vi "RT - Volume Track Math.vi"(10 "input cluster":T1={"Mute"=FALSE, "Solo"=FALSE, "Record"=FALSE, "Pan"=0.49531942166472487, "Volume"=0.0} {"Volume" scale=1.0..10.0; "Pan" scale=0.0..1.0}) -> (2 "Numeric":u16, 3 "Numeric 2":u16)   [LabVIEW 2014]
uses:
  Controls/Track Volume Settings.ctl
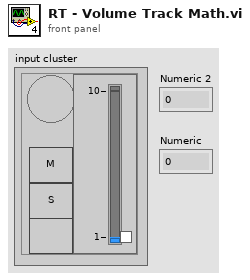
[diagram p1: front panel]
types:
  T1 = typedef "Track Volume Settings.ctl" = cluster{"Mute":bool, "Solo":bool, "Record":bool, "Pan":dbl, "Volume":dbl}
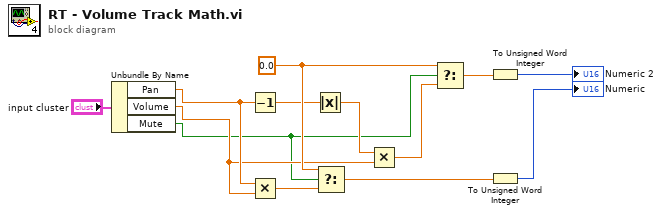
[diagram p0: block diagram]
diagram:
  w9 = 0.0 ("t")
  n1 = Unbundle By Name("input cluster") -> ("Pan"=w4:dbl, "Volume"=w3:dbl, "Mute"=w2:bool)
  n2 = Decrement(x=w4) -> (x-1=w5:dbl)
  n3 = Multiply(x=w4, y=w3) -> (x*y=w7:dbl)
  n4 = Absolute Value(x=w5) -> (abs(x)=w6:dbl)
  n5 = Select(t=w9, s=w2, f=w7) -> (s? t:f=w10:dbl)
  n6 = Multiply(x=w6, y=w3) -> (x*y=w8:dbl)
  n7 = Select(t=w9, s=w2, f=w8) -> (s? t:f=w11:dbl)
  n8 = To Unsigned Word Integer(number=w11) -> (unsigned 16bit integer=→"Numeric 2":u16)
  n9 = To Unsigned Word Integer(number=w10) -> (unsigned 16bit integer=→"Numeric":u16)
